vi "Pump Status.vi"(0 "ASIA Pump C Settings in":T2, 11 "error in (no error)":errorcluster) -> (1 "pressure":dbl, 3 "PumpStatusCode":T1(ring)=enum."Idle", 4 "ASIA Pump C Settings out":T2, 6 "Pump On?":enum16{"Off", "On", "Not Initialized"}(ring), 8 "Overpressure":bool, 10 "Connection Error":bool, 12 "syringeSize (ml)":sgl, 14 "pumpRate":dbl format="%.2f", 15 "error out":errorcluster)   [LabVIEW 2018, in "ASIA Pump.lvlib"]
uses:
  ASIA Pump.lvlib
  Pump Settings.ctl
  Program Files (x86)/Pfizer/FAST/data/AsiaPumpInterface.dll
panel:
  out "path out":path
  out "error":string
  out "Task Completed":u8
  out "pumpIndex":i32
  out "Error":string
  out "lastOverPressure":i32
  out "errorCode":i32
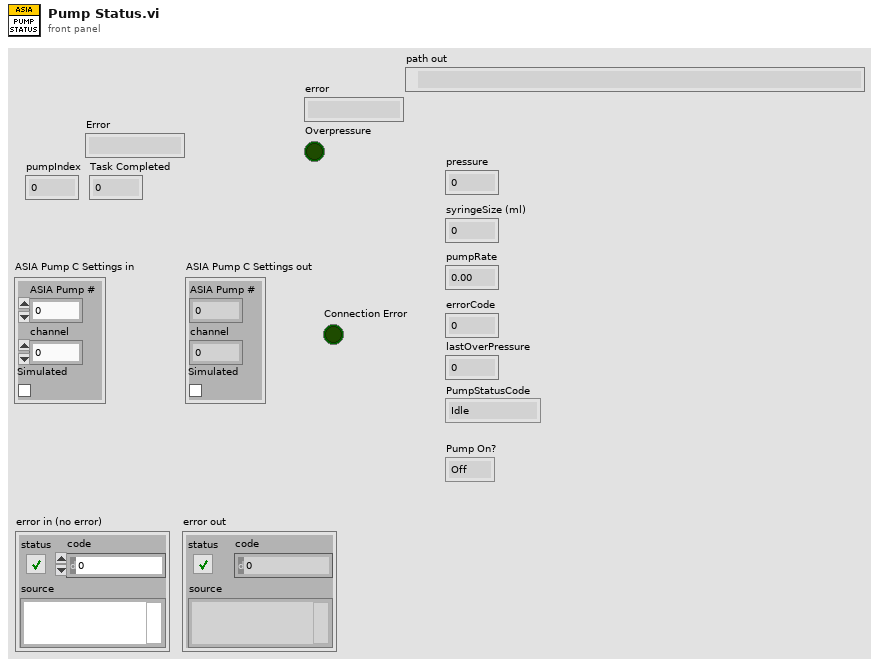
[diagram p1: front panel]
types:
  T1 = enum16{"Error", "Uninitialised", "Initialising", "Idle", "Filling", "Full", "Emptying", "Empty", "Pumping", "Default"}
  T2 = typedef "ASIA Pump.lvlib/Pump Settings.ctl" = cluster{"ASIA Pump #":i32, "channel":i32, "Simulated":bool}
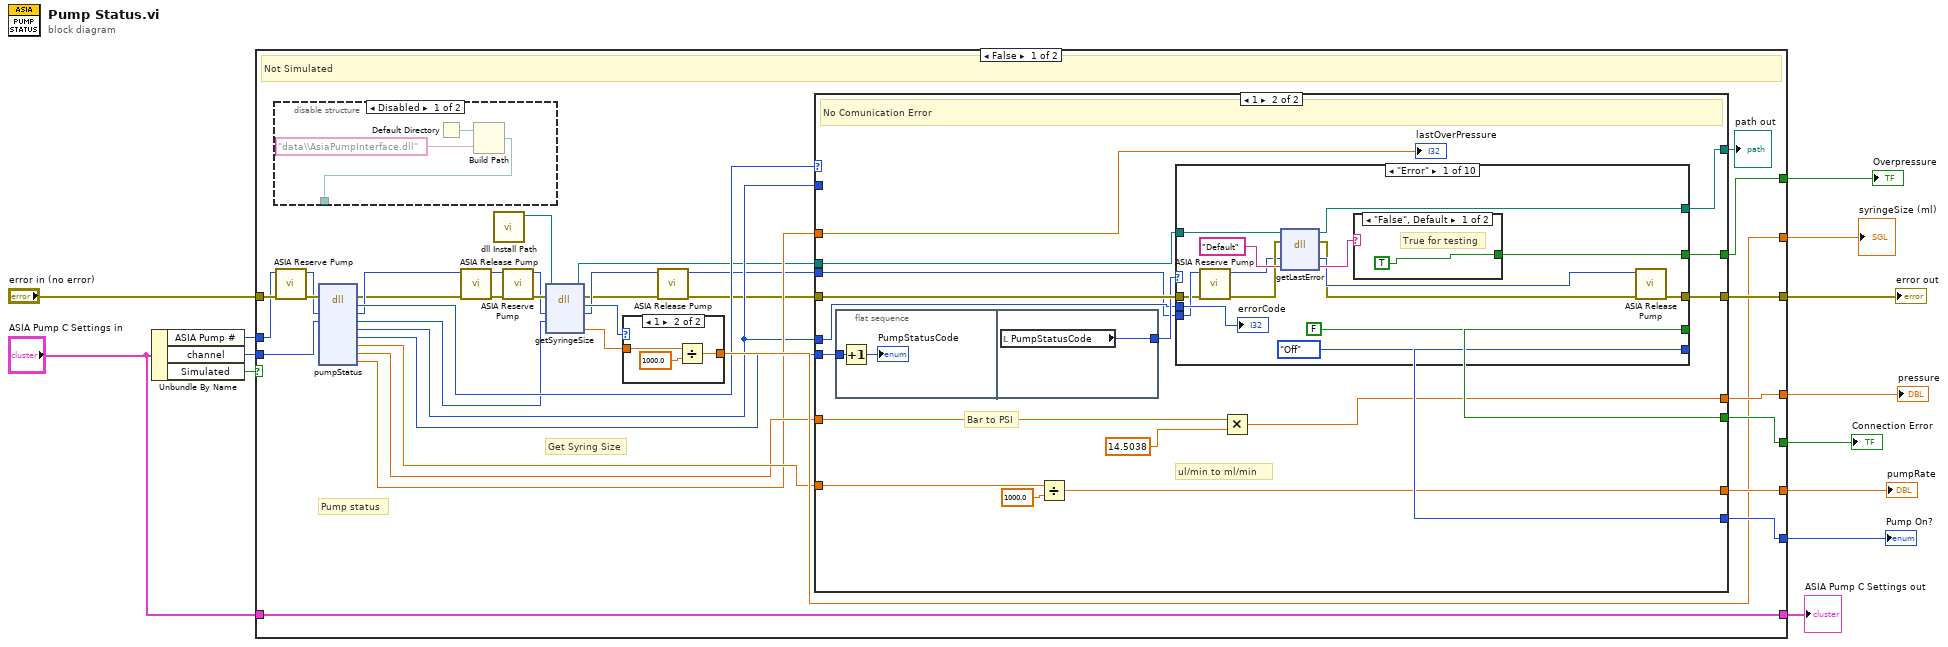
[diagram p0: block diagram]
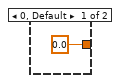
[diagram p3: hidden frame]
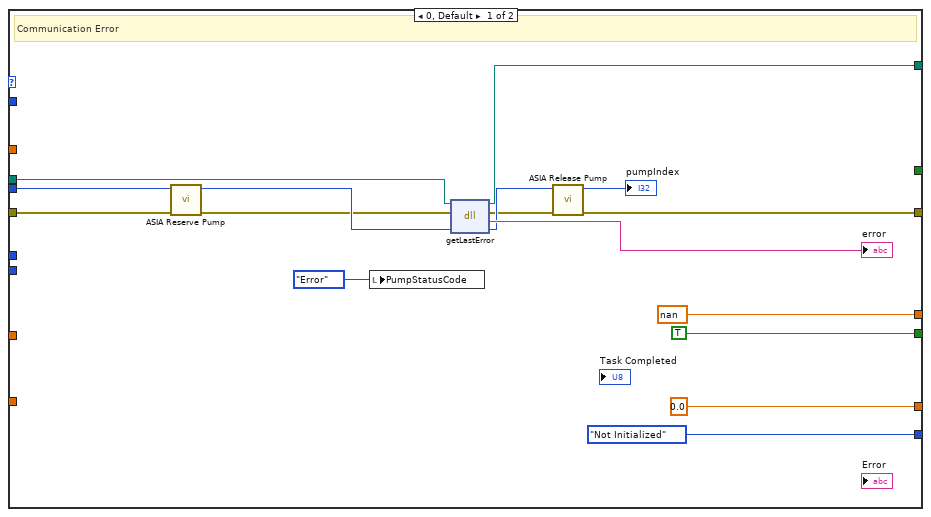
[diagram p4: hidden frame]
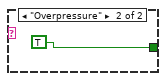
[diagram p5: hidden frame]
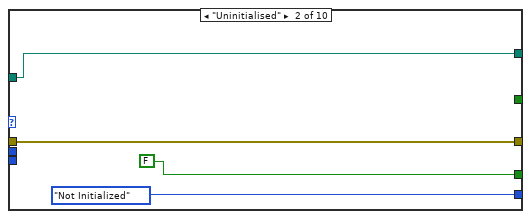
[diagram p6: hidden frame]
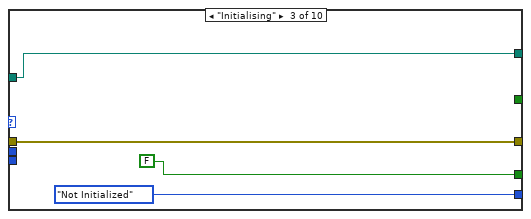
[diagram p7: hidden frame]
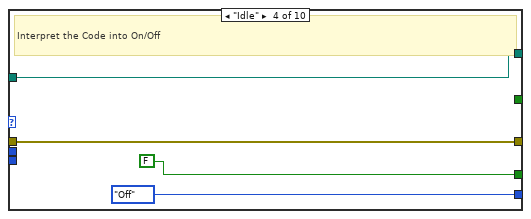
[diagram p8: hidden frame]
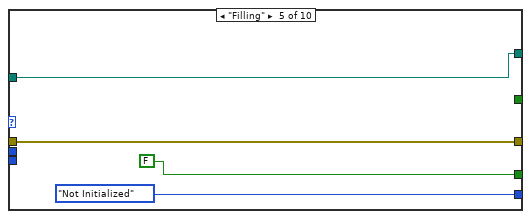
[diagram p9: hidden frame]
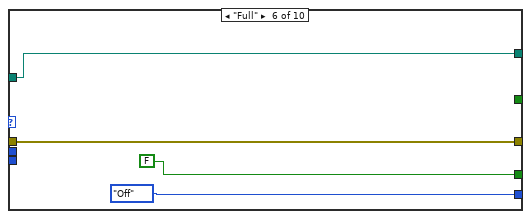
[diagram p10: hidden frame]
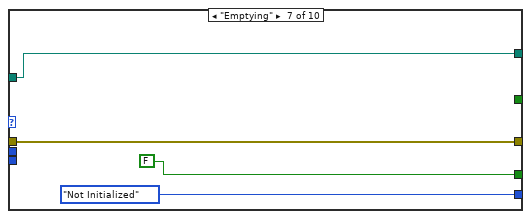
[diagram p11: hidden frame]
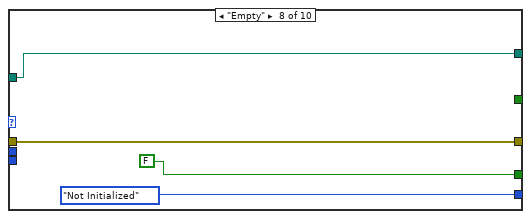
[diagram p12: hidden frame]
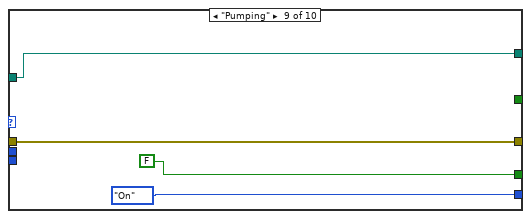
[diagram p13: hidden frame]
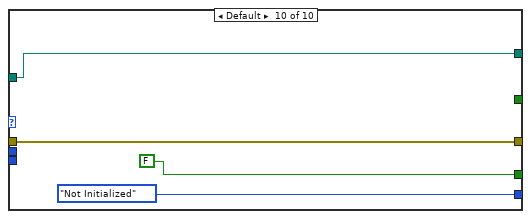
[diagram p14: hidden frame]
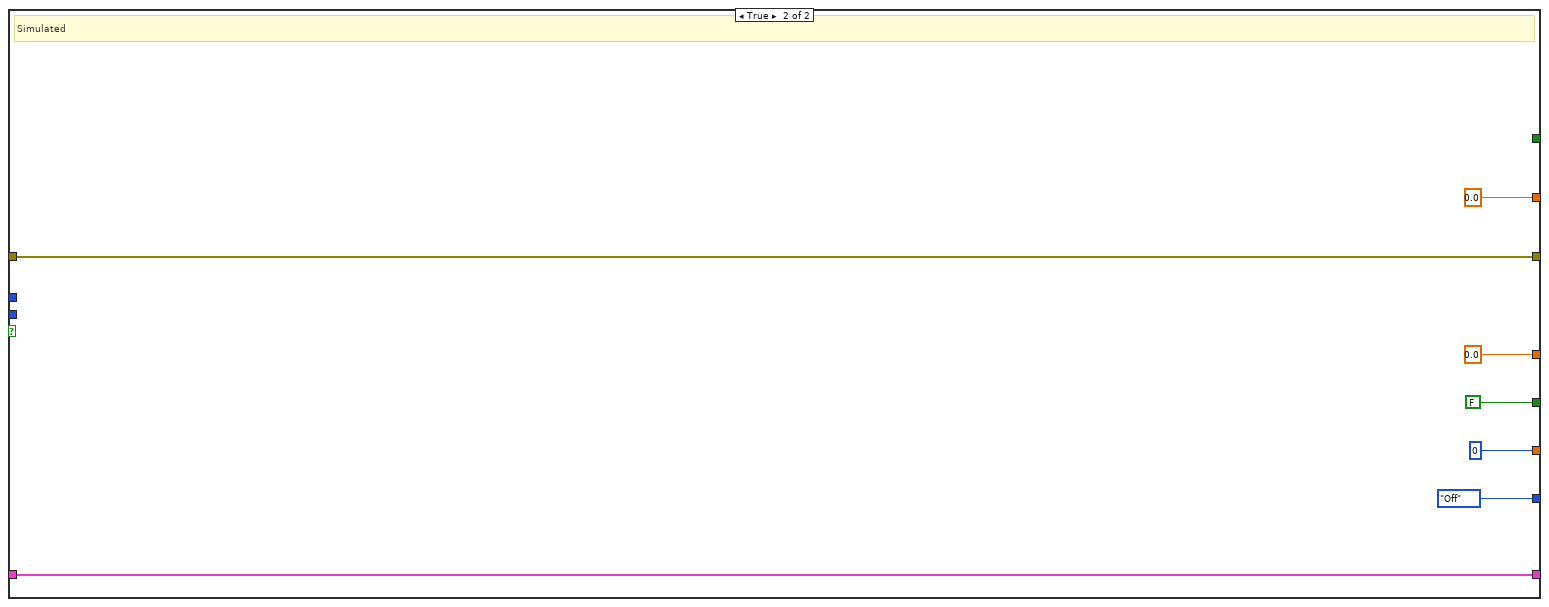
[diagram p15: hidden frame]
diagram:
  n1 = Unbundle By Name("ASIA Pump C Settings in") -> ("ASIA Pump #"=w2:i32, "channel"=w1:i32, "Simulated"=w3:bool)
  n2 = case shown="False" w3 {
    tunnel: [w48 FALSE ("Connection Error")] -> w13
    tunnel: [w47 w146] -> w12
    tunnel: [w46 0 ("pumpRate")] -> w11
    tunnel: [w45 enum16{"Off", "On", "Not Initialized"}."Off" ("Pump On?")] -> w10
    tunnel: [w40 sgl 0.0 ("syringeSize")] -> w9
    tunnel: [w42 sgl 0.0 ("pressure")] -> w8
    tunnel: "ASIA Pump C Settings in" -> [w41 w147]
    tunnel: [w41 w147] -> w6
    tunnel: "error in (no error)" -> [w32 w146]
    tunnel: w2 -> [w30 _]
    tunnel: w1 -> [w39 _]
    tunnel: [w25 _] -> w4
    frame False {
      # "Get Syring Size"
      # "Pump status"
      # "Not Simulated"
      n3 = disable-structure shown="Disabled" {
        disable-tunnel: [w49 _] -> _
        frame Disabled {
          n4 = Default Directory() -> (w50:path)
          n5 = Build Path(base path=w50, name or relative path="data\\AsiaPumpInterface.dll") -> (appended path=w49:path)
        }
        frame Enabled {
        }
      }
      n6 = call "ASIA Reserve Pump.vi"("error in (no error)"=w32, "ASIA Pump # In"=w30) -> ("error out"=w31:errorcluster, "ASIA Pump # Out"=w29:i32)  [unwired: 8 in]
      n7 = dll-call lib="C:/Program Files (x86)/Pfizer/FAST/data/AsiaPumpInterface.dll" fn="pumpStatus"(error in=w31, "pumpNum"=w29, "channel"=w39) -> (error out=w19:errorcluster, "Task Completed"=w38:u8, "pumpNum"=w20:u32, "channel"=w33:u32, "errorCode"=w26:i32, "pumpState"=w37:i32, "pumpRate"=w36:sgl, "pressure"=w35:sgl, "lastOverPressure"=w34:sgl)  [unwired: 7 in, 1 out]
      n8 = call "ASIA Release Pump.vi"("error in (no error)"=w19, "pumpNum"=w20) -> ("error out"=w18:errorcluster, "ASIA Pump # Out"=w17:i32)  [unwired: 8 in]
      n9 = call "dll Install Path.vi"() -> ("system directory"=w16:path)  [unwired: 11 in]
      n10 = call "ASIA Reserve Pump.vi"("error in (no error)"=w18, "ASIA Pump # In"=w17) -> ("error out"=w28:errorcluster, "ASIA Pump # Out"=w27:i32)  [unwired: 8 in]
      n11 = dll-call lib="C:/Program Files (x86)/Pfizer/FAST/data/AsiaPumpInterface.dll" fn="getSyringeSize"(path in=w16, error in=w28, "pumpNum"=w27, "channel"=w33) -> (path out=w15:path, error out=w23:errorcluster, "Task Completed"=w44:u8, "pumpNum"=w24:u32, "syringeSize"=w43:sgl)  [unwired: 3 in]
      n12 = case shown="1" w44 {
        tunnel: w43 -> [_ w54]
        tunnel: [sgl 0.0 ("syringeSize") w53] -> w40
        frame 0, Default {
        }
        frame 1 {
          n13 = Divide(x=w54, y=1000.0) -> (x/y=w53:dbl)
        }
      }
      n14 = call "ASIA Release Pump.vi"("error in (no error)"=w23, "pumpNum"=w24) -> ("error out"=w22:errorcluster, "ASIA Pump # Out"=w21:i32)  [unwired: 8 in]
      n15 = case shown="1" w38 {
        tunnel: [TRUE w89] -> w48
        tunnel: [w58 w88] -> w47
        tunnel: w22 -> [w65 w87]
        tunnel: w36 -> [_ w78]
        tunnel: w37 -> [_ w85]
        tunnel: w26 -> [_ _]
        tunnel: w35 -> [_ w81]
        tunnel: w34 -> [_ w86]
        tunnel: [0.0 ("pumpRate") w77] -> w46
        tunnel: [enum16{"Off", "On", "Not Initialized"}."Not Initialized" ("Pump On?") w83] -> w45
        tunnel: [sgl nan ("pressure") w80] -> w42
        tunnel: w21 -> [w64 w75]
        tunnel: w26 -> [_ w76]
        tunnel: [_ w74] -> w25
        tunnel: w15 -> [w57 w73]
        tunnel: [w56 w72] -> w14
        frame 0, Default {
          # "Communication Error"
          n16 = call "ASIA Reserve Pump.vi"("error in (no error)"=w65, "ASIA Pump # In"=w64) -> ("error out"=w62:errorcluster, "ASIA Pump # Out"=w63:i32)  [unwired: 8 in]
          n17 = local write "PumpStatusCode"(T1."Error" ("PumpStatusCode")) -> ()
          n18 = dll-call lib="C:/Program Files (x86)/Pfizer/FAST/data/AsiaPumpInterface.dll" fn="getLastError"(path in=w57, error in=w62, "pumpIndex"=w63) -> (path out=w56:path, error out=w59:errorcluster, "error"=→"error":string, "pumpIndex"=w61:i32)  [unwired: 1 in]
          n19 = call "ASIA Release Pump.vi"("error in (no error)"=w59, "pumpNum"=w61) -> ("error out"=w58:errorcluster, "ASIA Pump # Out"=→"pumpIndex":i32)  [unwired: 8 in]
        }
        frame 1 {
          # "ul/min to ml/min"
          # "Bar to PSI"
          # "No Comunication Error"
          n20 = flat-sequence {
            tunnel: w85 -> [w91]
            tunnel: [w92] -> w84
            frame #0 {
              n21 = Increment(x=w91) -> (x+1=→"PumpStatusCode":i32)
            }
            frame #1 {
              n22 = local read "PumpStatusCode"() -> (w92:T1)
            }
          }
          n23 = Divide(x=w78, y=1000.0) -> (x/y=w77:dbl)
          n24 = case shown="\"Error\"" w84 {
            tunnel: [FALSE FALSE FALSE FALSE FALSE FALSE FALSE FALSE FALSE FALSE] -> w89
            tunnel: w87 -> [w100 w112 w116 w120 w124 w128 w132 w136 w140 w144]
            tunnel: [w95 w112 w116 w120 w124 w128 w132 w136 w140 w144] -> w88
            tunnel: w75 -> [w101 _ _ _ _ _ _ _ _ _]
            tunnel: [enum16{"Off", "On", "Not Initialized"}."Off" ("Pump On?") enum16{"Off", "On", "Not Initialized"}."Not Initialized" ("Pump On?") enum16{"Off", "On", "Not Initialized"}."Not Initialized" ("Pump On?") enum16{"Off", "On", "Not Initialized"}."Off" ("Pump On?") enum16{"Off", "On", "Not Initialized"}."Not Initialized" ("Pump On?") enum16{"Off", "On", "Not Initialized"}."Off" ("Pump On?") enum16{"Off", "On", "Not Initialized"}."Not Initialized" ("Pump On?") enum16{"Off", "On", "Not Initialized"}."Not Initialized" ("Pump On?") enum16{"Off", "On", "Not Initialized"}."On" ("Pump On?") enum16{"Off", "On", "Not Initialized"}."Not Initialized" ("Pump On?")] -> w83
            tunnel: w76 -> [w105 _ _ _ _ _ _ _ _ _]
            tunnel: [w102 _ _ _ _ _ _ _ _ _] -> w74
            tunnel: w73 -> [w94 w110 w114 w118 w122 w126 w130 w134 w138 w142]
            tunnel: [w93 w110 w114 w118 w122 w126 w130 w134 w138 w142] -> w72
            frame "Error" {
              n25 = call "ASIA Reserve Pump.vi"("error in (no error)"=w100, "ASIA Pump # In"=w101) -> ("error out"=w99:errorcluster, "ASIA Pump # Out"=w98:i32)  [unwired: 8 in]
              n26 = dll-call lib="C:/Program Files (x86)/Pfizer/FAST/data/AsiaPumpInterface.dll" fn="getLastError"(path in=w94, error in=w99, "pumpNum"=w98, "Error"="Default") -> (path out=w93:path, error out=w96:errorcluster, "pumpNum"=w97:u32, "Error"=w103:string)  [unwired: 2 in]
              n27 = case shown="\"False\", Default" w103 {
                tunnel: [TRUE ("Overpressure") TRUE ("Overpressure")] -> w102
                frame "False", Default {
                  # "True for testing"
                }
                frame "Overpressure" {
                }
              }
              n28 = call "ASIA Release Pump.vi"("error in (no error)"=w96, "pumpNum"=w97) -> ("error out"=w95:errorcluster)  [unwired: 8 in, 1 out]
              "errorCode" <- w105
            }
            frame "Uninitialised" {
            }
            frame "Initialising" {
            }
            frame "Idle" {
              # "Interpret the Code into On/Off"
            }
            frame "Filling" {
            }
            frame "Full" {
            }
            frame "Emptying" {
            }
            frame "Empty" {
            }
            frame "Pumping" {
            }
            frame Default {
            }
          }
          n29 = Multiply(x=w81, y=14.5038) -> (x*y=w80:dbl)
          "lastOverPressure" <- w86
        }
      }
      "path out" <- w14
    }
    frame True {
      # "Simulated"
    }
  }
  "error out" <- w12
  "ASIA Pump C Settings out" <- w6
  "Connection Error" <- w13
  "pumpRate" <- w11
  "Pump On?" <- w10
  "syringeSize (ml)" <- w9
  "pressure" <- w8
  "Overpressure" <- w4
